vi "WhereGo.vi"(7 "QR CODE":bool, 8 "Block Array":dbl[][](array[numeric]), 9 "Catch Color":dbl[](array[numeric]), 10 "Put Counter":i16, 11 "Block Color":dbl[][](array[numeric])) -> (0 "Block Array Out":dbl[][](array[numeric]), 2 "Proc Block Index":i16)   [LabVIEW 2018]
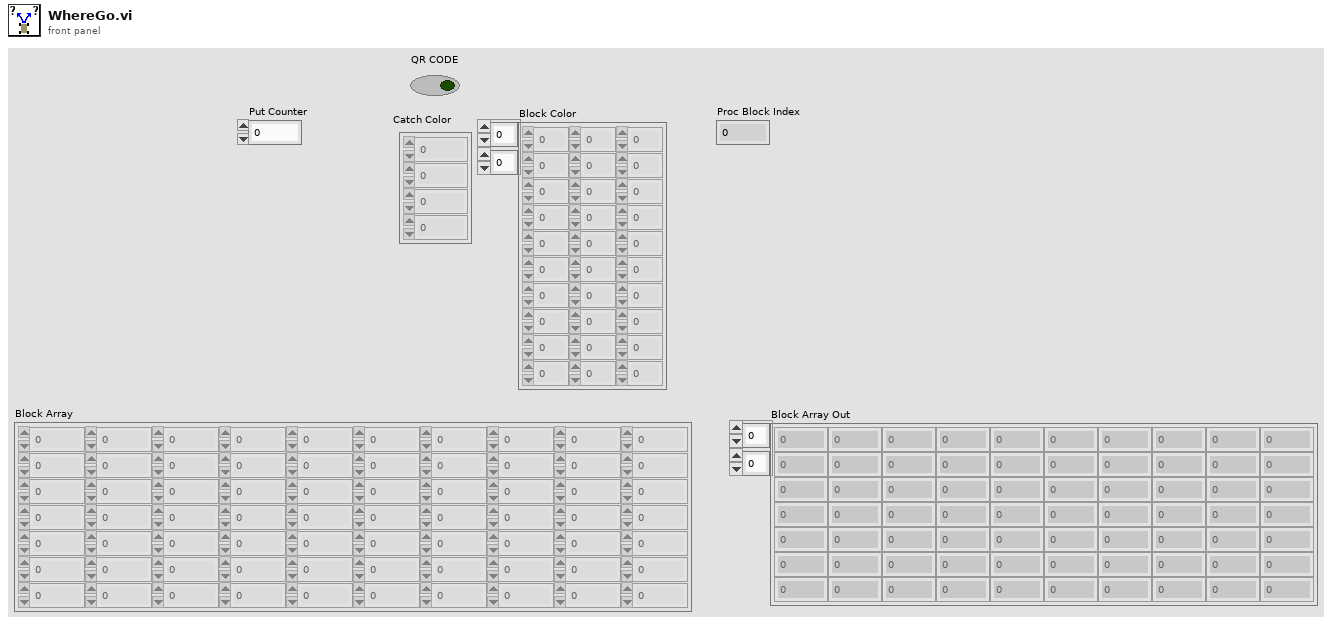
[diagram p1: front panel]
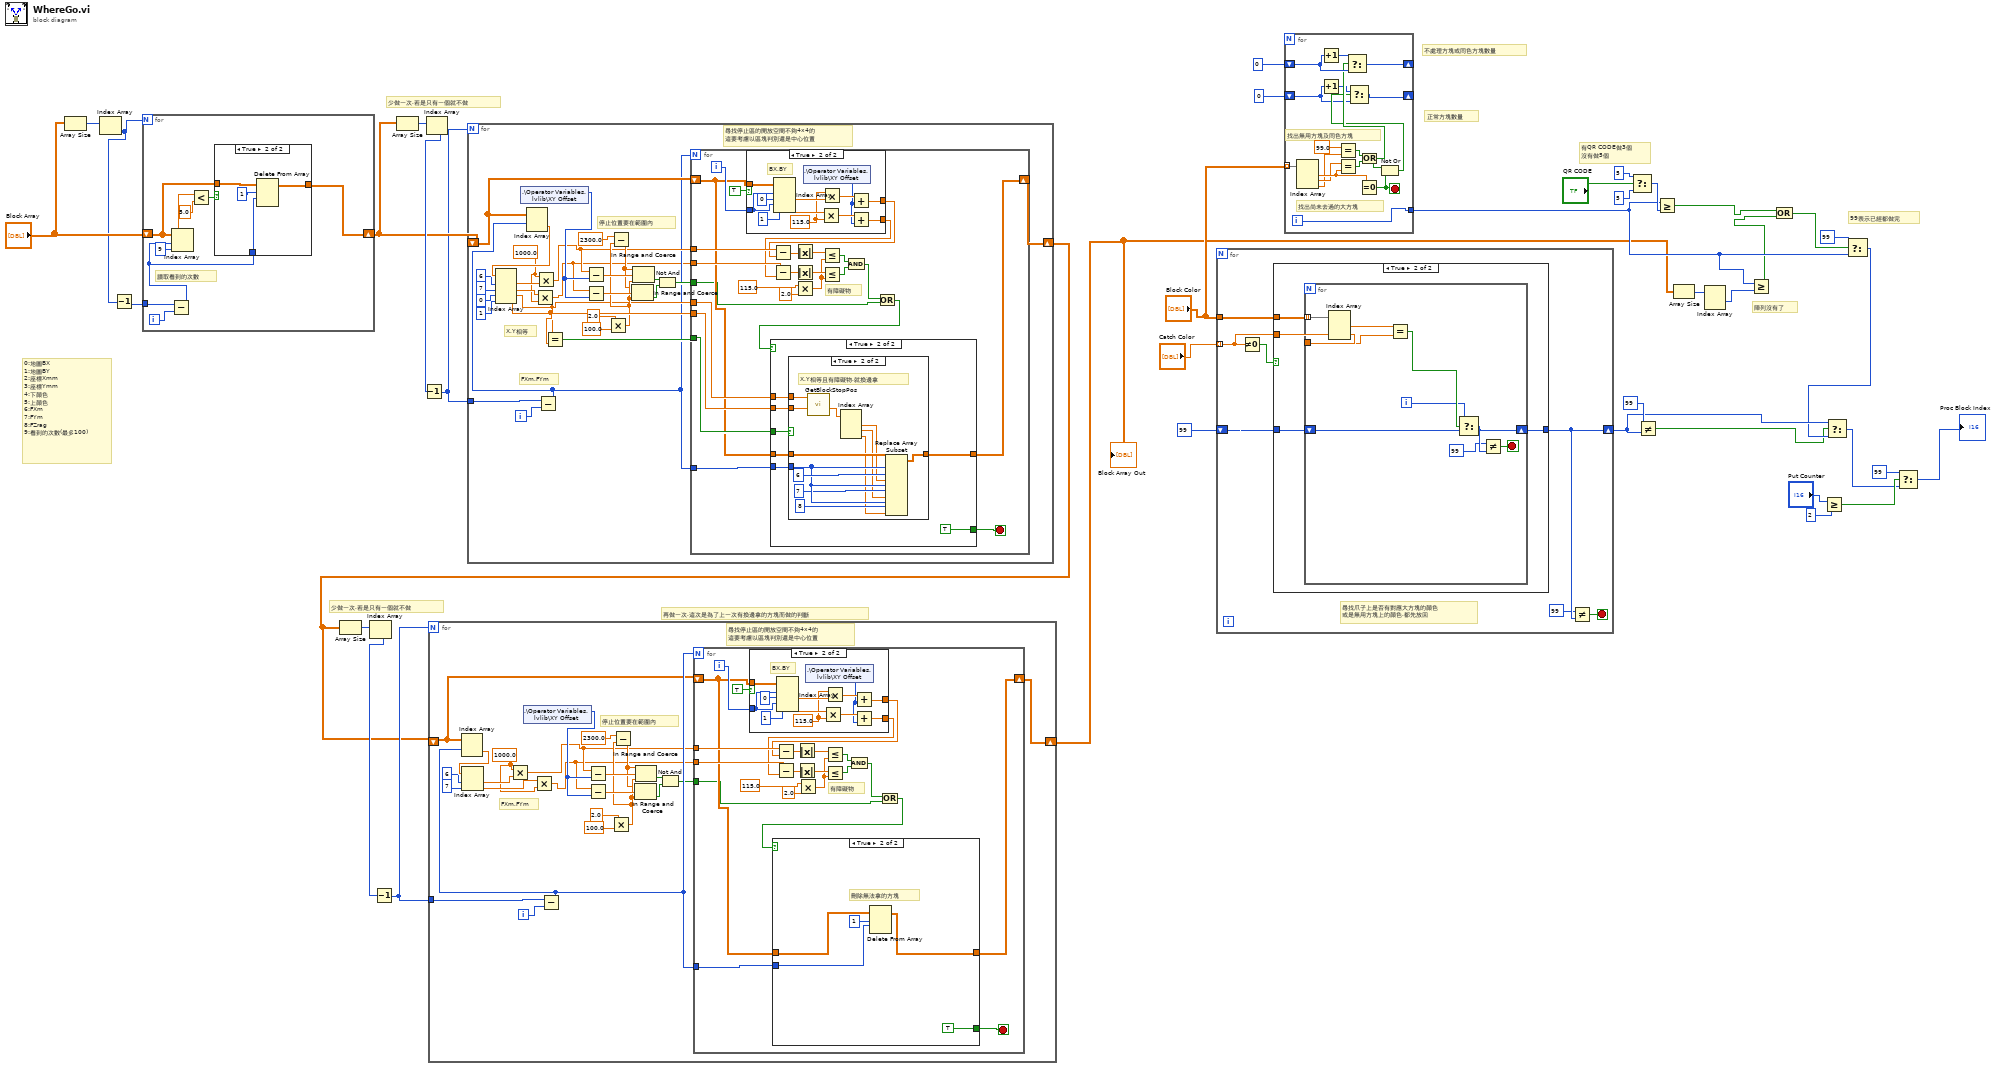
[diagram p0: block diagram]
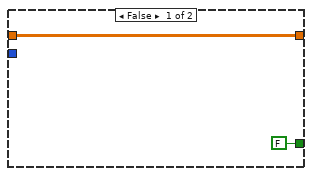
[diagram p2: hidden frame]
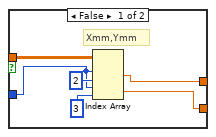
[diagram p3: hidden frame]
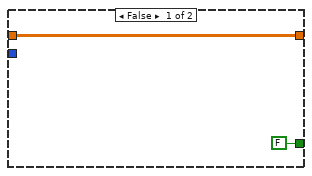
[diagram p4: hidden frame]
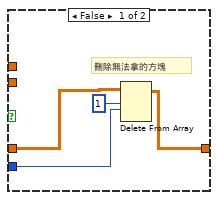
[diagram p5: hidden frame]
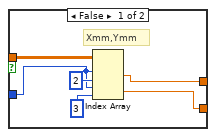
[diagram p6: hidden frame]
diagram:
  # "再做一次,這次是為了上一次有換邊拿的方塊而做的判斷"
  # "少做一次,若是只有一個就不做"
  # "少做一次,若是只有一個就不做"
  # "0:地圖BX\n1:地圖BY\n2:座標Xmm\n3:座標Ymm\n4:下顏色\n5:上顏色\n6:FXm\n7:FYm\n8:FZrag\n9:看到的次數(最多100)"
  # "陣列沒有了"
  # "正常方塊數量"
  # "不處理方塊或同色方塊數量"
  # "有QR CODE做3個\n沒有做5個"
  # "99表示已經都做完"
  n1 = Array Size(array="Block Array") -> (size(s)=w23:i32[])
  n2 = Index Array(array=w23) -> (element=w21:i32)  [unwired: 1 in]
  n3 = Decrement(x=w21) -> (x-1=w20:i32)
  n4 = for {
    N: w21 -> [_]
    tunnel: w20 -> [w47]
    shift-right: [w40] -> w17
    shift-left: "Block Array" -> [w45]
    i -> [w48]
    # "讀取看到的次數"
    n5 = Subtract(x=w47, y=w48) -> (x-y=w41:i32)
    n6 = Index Array(array=w45, index (row)=w41, index (col)=9 ("disabled index (col)")) -> (element=w43:dbl)
    n7 = Less?(x=w43, y=5.0) -> (x < y?=w44:bool)
    n8 = case shown="True" w44 {
      tunnel: w45 -> [w49 w53]
      tunnel: w41 -> [_ w51]
      tunnel: [w49 w50] -> w40
      frame False {
      }
      frame True {
        n9 = Delete From Array(array=w53, length=1, index (row)=w51) -> (array with subset deleted=w50:dbl[][])  [unwired: 1 in, 1 out]
      }
    }
  }
  n10 = Array Size(array=w17) -> (size(s)=w18:i32[])
  n11 = Index Array(array=w18) -> (element=w19:i32)  [unwired: 1 in]
  n12 = Decrement(x=w19) -> (x-1=w16:i32)
  n13 = for {
    N: w16 -> [_]
    tunnel: w16 -> [w81]
    shift-right: [w73] -> w12
    shift-left: w17 -> [w80]
    i -> [w82]
    w55 = 1000.0 ("x")
    # "停止位置要在範圍內"
    # "X,Y相等"
    # "尋找停止區的開放空間不夠4x4的\n這要考慮以區塊判別還是中心位置"
    # "FXm,FYm"
    n14 = shared-variable ".\\Operator Variables.lvlib\\XY Offset"() -> (w65:i16)  [unwired: 1 in, 1 out]
    n15 = Subtract(x=w81, y=w82) -> (x-y=w56:i32)
    n16 = Index Array(array=w80, index (row)=w56) -> (element=w79:dbl[])  [unwired: 1 in]
    n17 = Index Array(array=w79, index #1=6 ("index"), index #2=7 ("index"), index #3=0 ("index"), index #4=1 ("index")) -> (element #1=w60:dbl, element #2=w57:dbl, element #3=w58:dbl, element #4=w72:dbl)
    n18 = Multiply(x=w57, y=w55) -> (x*y=w54:dbl)
    n19 = Multiply(x=w55, y=w60) -> (x*y=w59:dbl)
    n20 = Equal?(x=w58, y=w72) -> (x = y?=w74:bool)
    n21 = Subtract(x=w59, y=w65) -> (x-y=w71:dbl)
    n22 = Subtract(x=w54, y=w65) -> (x-y=w70:dbl)
    n23 = Multiply(x=2.0, y=100.0 ("lower limit")) -> (x*y=w66:dbl)
    n24 = Subtract(x=2300.0 ("lower limit"), y=w66) -> (x-y=w61:dbl)
    n25 = In Range and Coerce(upper limit=w61, x=w70, lower limit=w66) -> (In Range?=w63:bool)  [unwired: 1 out]
    n26 = In Range and Coerce(upper limit=w61, x=w71, lower limit=w66) -> (In Range?=w64:bool)  [unwired: 1 out]
    n27 = Not And(1:w63, 2:w64) -> (0:w62:bool)
    n28 = for {
      N: w56 -> [_]
      tunnel: w59 -> [w106]
      tunnel: w54 -> [w105]
      tunnel: w74 -> [w94]
      tunnel: w58 -> [w93]
      tunnel: w72 -> [w92]
      shift-right: [w90] -> w73
      shift-left: w80 -> [w91]
      tunnel: w56 -> [w89]
      tunnel: w62 -> [w84]
      i -> [w107]
      stop <- w88 stop-if-true
      # "有障礙物"
      n29 = case shown="True" TRUE {
        tunnel: w91 -> [w133 w148]
        tunnel: w107 -> [w136 w147]
        tunnel: [w135 w140] -> w86
        tunnel: [w134 w139] -> w87
        frame False {
          # "Xmm,Ymm"
          n30 = Index Array(array=w133, index (row) #1=w136, index (col) #1=2 ("disabled index (col)"), index (row) #2=w136, index (col) #2=3 ("disabled index (col)")) -> (element #1=w135:dbl, element #2=w134:dbl)
        }
        frame True {
          w144 = 115.0 ("y")
          # "BX,BY"
          n31 = Index Array(array=w148, index (row) #1=w147, index (col) #1=0 ("disabled index (col)"), index (row) #2=w147, index (col) #2=1 ("disabled index (col)")) -> (element #1=w145:dbl, element #2=w146:dbl)
          n32 = shared-variable ".\\Operator Variables.lvlib\\XY Offset"() -> (w141:i16)  [unwired: 1 in, 1 out]
          n33 = Multiply(x=w146, y=w144) -> (x*y=w142:dbl)
          n34 = Multiply(x=w144, y=w145) -> (x*y=w143:dbl)
          n35 = Add(x=w143, y=w141) -> (x+y=w140:dbl)
          n36 = Add(x=w142, y=w141) -> (x+y=w139:dbl)
        }
      }
      n37 = Subtract(x=w106, y=w86) -> (x-y=w104:dbl)
      n38 = Subtract(x=w105, y=w87) -> (x-y=w103:dbl)
      n39 = Absolute Value(x=w104) -> (abs(x)=w102:dbl)
      n40 = Absolute Value(x=w103) -> (abs(x)=w101:dbl)
      n41 = Multiply(x=115.0 ("y"), y=2.0) -> (x*y=w98:dbl)
      n42 = Less Or Equal?(x=w102, y=w98) -> (x <= y?=w97:bool)
      n43 = Less Or Equal?(x=w101, y=w98) -> (x <= y?=w96:bool)
      n44 = And(x=w97, y=w96) -> (x .and. y?=w85:bool)
      n45 = Or(x=w85, y=w84) -> (x .or. y?=w83:bool)
      n46 = case shown="True" w83 {
        tunnel: w94 -> [_ w116]
        tunnel: w93 -> [_ w115]
        tunnel: w92 -> [_ w114]
        tunnel: w91 -> [w109 w113]
        tunnel: [w109 w111] -> w90
        tunnel: w89 -> [_ w112]
        tunnel: [FALSE TRUE] -> w88
        frame False {
        }
        frame True {
          n47 = case shown="True" w116 {
            tunnel: w115 -> [_ w132]
            tunnel: w114 -> [_ w131]
            tunnel: w113 -> [w119 w130]
            tunnel: w112 -> [w118 w127]
            tunnel: [w117 w121] -> w111
            frame False {
              # "刪除無法拿的方塊"
              n48 = Delete From Array(array=w119, length=1, index (row)=w118) -> (array with subset deleted=w117:dbl[][])  [unwired: 1 in, 1 out]
            }
            frame True {
              # "X,Y相等且有障礙物,就換邊拿"
              n49 = call "GetBlockStopPos.vi"("YB"=w131, "XB"=w132) -> ("Array B"=w125:dbl[])  [unwired: 8 in, 1 out]
              n50 = Index Array(array=w125) -> (element #1=w124:dbl, element #2=w123:dbl, element #3=w122:dbl)  [unwired: 3 in]
              n51 = Replace Array Subset(array=w130, new element #1=w124, index (row) #1=w127, index (col) #1=6 ("disabled index (col)"), new element #2=w123, index (row) #2=w127, index (col) #2=7 ("disabled index (col)"), new element #3=w122, index (row) #3=w127, index (col) #3=8 ("disabled index (col)")) -> (w121:dbl[][])
            }
          }
        }
      }
    }
  }
  n52 = Array Size(array=w12) -> (size(s)=w14:i32[])
  n53 = Index Array(array=w14) -> (element=w13:i32)  [unwired: 1 in]
  n54 = Decrement(x=w13) -> (x-1=w15:i32)
  n55 = for {
    N: w15 -> [_]
    tunnel: w15 -> [w173]
    shift-right: [w169] -> w11
    shift-left: w12 -> [w156]
    i -> [w174]
    w151 = 1000.0 ("x")
    # "停止位置要在範圍內"
    # "尋找停止區的開放空間不夠4x4的\n這要考慮以區塊判別還是中心位置"
    # "FXm,FYm"
    n56 = shared-variable ".\\Operator Variables.lvlib\\XY Offset"() -> (w161:i16)  [unwired: 1 in, 1 out]
    n57 = Subtract(x=w173, y=w174) -> (x-y=w168:i32)
    n58 = Index Array(array=w156, index (row)=w168) -> (element=w172:dbl[])  [unwired: 1 in]
    n59 = Index Array(array=w172, index #1=6 ("index"), index #2=7 ("index")) -> (element #1=w155:dbl, element #2=w153:dbl)
    n60 = Multiply(x=w151, y=w155) -> (x*y=w154:dbl)
    n61 = Multiply(x=w153, y=w151) -> (x*y=w152:dbl)
    n62 = Subtract(x=w154, y=w161) -> (x-y=w167:dbl)
    n63 = Subtract(x=w152, y=w161) -> (x-y=w166:dbl)
    n64 = Multiply(x=2.0, y=100.0 ("lower limit")) -> (x*y=w162:dbl)
    n65 = Subtract(x=2300.0 ("lower limit"), y=w162) -> (x-y=w157:dbl)
    n66 = In Range and Coerce(upper limit=w157, x=w166, lower limit=w162) -> (In Range?=w159:bool)  [unwired: 1 out]
    n67 = In Range and Coerce(upper limit=w157, x=w167, lower limit=w162) -> (In Range?=w160:bool)  [unwired: 1 out]
    n68 = Not And(1:w159, 2:w160) -> (0:w158:bool)
    n69 = for {
      N: w168 -> [_]
      tunnel: w154 -> [w195]
      tunnel: w152 -> [w194]
      shift-right: [w182] -> w169
      shift-left: w156 -> [w183]
      tunnel: w168 -> [w181]
      tunnel: w158 -> [w176]
      i -> [w196]
      stop <- w180 stop-if-true
      # "有障礙物"
      n70 = case shown="True" TRUE {
        tunnel: w183 -> [w204 w219]
        tunnel: w196 -> [w207 w218]
        tunnel: [w206 w211] -> w178
        tunnel: [w205 w210] -> w179
        frame False {
          # "Xmm,Ymm"
          n71 = Index Array(array=w204, index (row) #1=w207, index (col) #1=2 ("disabled index (col)"), index (row) #2=w207, index (col) #2=3 ("disabled index (col)")) -> (element #1=w206:dbl, element #2=w205:dbl)
        }
        frame True {
          w215 = 115.0 ("y")
          # "BX,BY"
          n72 = Index Array(array=w219, index (row) #1=w218, index (col) #1=0 ("disabled index (col)"), index (row) #2=w218, index (col) #2=1 ("disabled index (col)")) -> (element #1=w216:dbl, element #2=w217:dbl)
          n73 = shared-variable ".\\Operator Variables.lvlib\\XY Offset"() -> (w212:i16)  [unwired: 1 in, 1 out]
          n74 = Multiply(x=w217, y=w215) -> (x*y=w213:dbl)
          n75 = Multiply(x=w215, y=w216) -> (x*y=w214:dbl)
          n76 = Add(x=w214, y=w212) -> (x+y=w211:dbl)
          n77 = Add(x=w213, y=w212) -> (x+y=w210:dbl)
        }
      }
      n78 = Subtract(x=w195, y=w178) -> (x-y=w193:dbl)
      n79 = Subtract(x=w194, y=w179) -> (x-y=w192:dbl)
      n80 = Absolute Value(x=w193) -> (abs(x)=w191:dbl)
      n81 = Absolute Value(x=w192) -> (abs(x)=w190:dbl)
      n82 = Multiply(x=115.0 ("y"), y=2.0) -> (x*y=w187:dbl)
      n83 = Less Or Equal?(x=w191, y=w187) -> (x <= y?=w186:bool)
      n84 = Less Or Equal?(x=w190, y=w187) -> (x <= y?=w185:bool)
      n85 = And(x=w186, y=w185) -> (x .and. y?=w177:bool)
      n86 = Or(x=w177, y=w176) -> (x .or. y?=w175:bool)
      n87 = case shown="True" w175 {
        tunnel: w183 -> [w198 w203]
        tunnel: [w198 w201] -> w182
        tunnel: w181 -> [_ w202]
        tunnel: [FALSE TRUE] -> w180
        frame False {
        }
        frame True {
          # "刪除無法拿的方塊"
          n88 = Delete From Array(array=w203, length=1, index (row)=w202) -> (array with subset deleted=w201:dbl[][])  [unwired: 1 in, 1 out]
        }
      }
    }
  }
  "Block Array Out" <- w11
  n89 = for {
    tunnel: "Catch Color" -> [w226] mode=indexing
    tunnel: "Block Color" -> [w227]
    shift-right: [w223] -> w28
    shift-left: 99 -> [w225]
    stop <- w224 stop-if-true
    # "尋找爪子上是否有對應大方塊的顏色\n或是無用方塊上的顏色,都先放回"
    n90 = Not Equal To 0?(x=w226) -> (x != 0?=w228:bool)
    n91 = case shown="True" w228 {
      tunnel: w227 -> [_ w233]
      tunnel: w226 -> [_ w232]
      tunnel: w225 -> [w229 w231]
      tunnel: [w229 w230] -> w223
      frame False {
      }
      frame True {
        n92 = for {
          tunnel: w233 -> [w242] mode=indexing
          tunnel: w232 -> [w236]
          shift-right: [w240] -> w230
          shift-left: w231 -> [w238]
          i -> [w234]
          stop <- w241 stop-if-true
          n93 = Index Array(array=w242) -> (element #1=w237:dbl)  [unwired: 3 in, 2 out]
          n94 = Equal?(x=w237, y=w236) -> (x = y?=w235:bool)
          n95 = Select(t=w234, s=w235, f=w238) -> (s? t:f=w240:i32)
          n96 = Not Equal?(x=99, y=w240) -> (x != y?=w241:bool)
        }
      }
    }
    n97 = Not Equal?(x=99, y=w223) -> (x != y?=w224:bool)
  }
  n98 = for {
    tunnel: "Block Color" -> [w259] mode=indexing
    tunnel: [w258] -> w25
    shift-right: [w249] -> _
    shift-left: 0 -> [w250]
    shift-right: [w243] -> _
    shift-left: 0 -> [w244]
    i -> [w258]
    stop <- w247 stop-if-true
    # "找出無用方塊及同色方塊"
    # "找出尚未去過的大方塊"
    n99 = Index Array(array=w259) -> (element #1=w257:dbl, element #2=w256:dbl, element #3=w255:dbl)  [unwired: 3 in]
    n100 = Increment(x=w250) -> (x+1=w251:i32)
    n101 = Increment(x=w244) -> (x+1=w245:i32)
    n102 = Equal?(x=w256, y=w257) -> (x = y?=w253:bool)
    n103 = Equal?(x=99.0, y=w255) -> (x = y?=w252:bool)
    n104 = Or(x=w252, y=w253) -> (x .or. y?=w248:bool)
    n105 = Select(t=w251, s=w248, f=w250) -> (s? t:f=w249:i32)
    n106 = Equal To 0?(x=w257) -> (x = 0?=w247:bool)
    n107 = Not Or(1:w247, 2:w248) -> (0:w246:bool)
    n108 = Select(t=w245, s=w246, f=w244) -> (s? t:f=w243:i32)
  }
  n109 = Select(t=5, s="QR CODE", f=5) -> (s? t:f=w32:i32)
  n110 = Not Equal?(x=99, y=w28) -> (x != y?=w5:bool)
  n111 = Greater Or Equal?(x=w25, y=w32) -> (x >= y?=w9:bool)
  n112 = Array Size(array=w11) -> (size(s)=w26:i32[])
  n113 = Index Array(array=w26) -> (element #1=w24:i32)  [unwired: 2 in, 1 out]
  n114 = Greater Or Equal?(x=w25, y=w24) -> (x >= y?=w10:bool)
  n115 = Compound Arithmetic op=OR(w9, w10) -> (w6:bool)
  n116 = Greater Or Equal?(x="Put Counter", y=i16 2) -> (x >= y?=w4:bool)
  n117 = Select(t=99, s=w6, f=w25) -> (s? t:f=w27:i32)
  n118 = Select(t=w28, s=w5, f=w27) -> (s? t:f=w3:i32)
  n119 = Select(t=99, s=w4, f=w3) -> (s? t:f=→"Proc Block Index":i32)
